vi "LoopselFF_1_or_2cam_eventdriven.VI"() -> ()   [LabVIEW 2015]
uses:
  board.vis/Globals.vi
  <vilib>/Analysis/NI_AALBase.lvlib
panel:
  out "tRMS":dbl=8.272957184592048 format="%0#.1f"
  out "mean":dbl=3064.5285285285286 format="%#_4f"
  in  "Pixel":u16=100
  in  "continuous":bool=TRUE
  out "curr.block":dbl=1.0
  out "Measure ON":bool
  in  "cam select\n1: cam 1\n2: cam 2\n3: both cams":u8=3
  in  "no.of blocks (nob)\npress enter":u32=1
  in  "NOB":u32(slide)=1 max=10 scale=0.9..1.0
  out "Signalverlaufgraph 2":u16[](graph)=[0, 0, 543, 543, 0, 1, 0, 0, 2, 2, 3, 3, 4, 4, 5, 5, 6, 6, 7, 7, 8, 8, 9, 9, 10, 10, 11, 11, 12, 12, 13, 13, 14, 14, 15, 15, 16, 16, 17, 17, 18, 18, 19, 19, 20, 20, 21, 21, 22, 22, 23, 23, 24, 24, 25, 25, 26, 26, 27, 27, 28, 28, 29, 29, 30, 30, 31, 31, 32, 32, 33, 33, 34, 34, 35, 35, 36, 36, 37, 37, 38, 38, 39, 39, 40, 40, 41, 41, 42, 42, 43, 43, 44, 44, 45, 45, 46, 46, 47, 47, 48, 48, 49, 49, 50, 50, 51, 51, 52, 52, 53, 53, 54, 54, 55, 55, 56, 56, 57, 57, 58, 58, 59, 59, 60, 60, 61, 61, 62, 62, 63, 63, 64, 64, 65, 65, 66, 66, 67, 67, 68, 68, 69, 69, 70, 70, 71, 71, 72, 72, 73, 73, 74, 74, 75, 75, 76, 76, 77, 77, 78, 78, 79, 79, 80, 80, 81, 81, 82, 82, 83, 83, 84, 84, 85, 85, 86, 86, 87, 87, 88, 88, 89, 89, 90, 90, 91, 91, 92, 92, 93, 93, 94, 94, 95, 95, 96, 96, 97, 97, 98, 98, 99, 99, 100, 100, 101, 101, 102, 102, 103, 103, 104, 104, 105, 105, 106, 106, 107, 107, 108, 108, 109, 109, 110, 110, 111, 111, 112, 112, 113, 113, 114, 114, 115, 115, 116, 116, 117, 117, 118, 118, 119, 119, 120, 120, 121, 121, 122, 122, 123, 123, 124, 124, 125, 125, 126, 126, 127, 127, 128, 128, 129, 129, 130, 130, 131, 131, 132, 132, 133, 133, 134, 134, 135, 135, 136, 136, 137, 137, 138, 138, 139, 139, 140, 140, 141, 141, 142, 142, 143, 143, 144, 144, 145, 145, 146, 146, 147, 147, 148, 148, 149, 149, 150, 150, 151, 151, 152, 152, 153, 153, 154, 154, 155, 155, 156, 156, 157, 157, 158, 158, 159, 159, 160, 160, 161, 161, 162, 162, 163, 163, 164, 164, 165, 165, 166, 166, 167, 167, 168, 168, 169, 169, 170, 170, 171, 171, 172, 172, 173, 173, 174, 174, 175, 175, 176, 176, 177, 177, 178, 178, 179, 179, 180, 180, 181, 181, 182, 182, 183, 183, 184, 184, 185, 185, 186, 186, 187, 187, 188, 188, 189, 189, 190, 190, 191, 191, 192, 192, 193, 193, 194, 194, 195, 195, 196, 196, 197, 197, 198, 198, 199, 199, 200, 200, 201, 201, 202, 202, 203, 203, 204, 204, 205, 205, 206, 206, 207, 207, 208, 208, 209, 209, 210, 210, 211, 211, 212, 212, 213, 213, 214, 214, 215, 215, 216, 216, 217, 217, 218, 218, 219, 219, 220, 220, 221, 221, 222, 222, 223, 223, 224, 224, 225, 225, 226, 226, 227, 227, 228, 228, 229, 229, 230, 230, 231, 231, 232, 232, 233, 233, 234, 234, 235, 235, 236, 236, 237, 237, 238, 238, 239, 239, 240, 240, 241, 241, 242, 242, 243, 243, 244, 244, 245, 245, 246, 246, 247, 247, 248, 248, 249, 249, 250, 250, 251, 251, 252, 252, 253, 253, 254, 254, 255, 255, 256, 256, 257, 257, 258, 258, 259, 259, 260, 260, 261, 261, 262, 262, 263, 263, 264, 264, 265, 265, 266, 266, 267, 267, 268, 268, 269, 269, 270, 270, 271, 271, 272, 272, 273, 273, 274, 274, 275, 275, 276, 276, 277, 277, 278, 278, 279, 279, 280, 280, 281, 281, 282, 282, 283, 283, 284, 284, 285, 285, 286, 286, 287, 287, 288, 288, 289, 289, 290, 290, 291, 291, 292, 292, 293, 293, 294, 294, 295, 295, 296, 296, 297, 297, 298, 298, 299, 299, 300, 300, 301, 301, 302, 302, 303, 303, 304, 304, 305, 305, 306, 306, 307, 307, 308, 308, 309, 309, 310, 310, 311, 311, 312, 312, 313, 313, 314, 314, 315, 315, 316, 316, 317, 317, 318, 318, 319, 319, 320, 320, 321, 321, 322, 322, 323, 323, 324, 324, 325, 325, 326, 326, 327, 327, 328, 328, 329, 329, 330, 330, 331, 331, 332, 332, 333, 333, 334, 334, 335, 335, 336, 336, 337, 337, 338, 338, 339, 339, 340, 340, 341, 341, 342, 342, 343, 343, 344, 344, 345, 345, 346, 346, 347, 347, 348, 348, 349, 349, 350, 350, 351, 351, 352, 352, 353, 353, 354, 354, 355, 355, 356, 356, 357, 357, 358, 358, 359, 359, 360, 360, 361, 361, 362, 362, 363, 363, 364, 364, 365, 365, 366, 366, 367, 367, 368, 368, 369, 369, 370, 370, 371, 371, 372, 372, 373, 373, 374, 374, 375, 375, 376, 376, 377, 377, 378, 378, 379, 379, 380, 380, 381, 381, 382, 382, 383, 383, 384, 384, 385, 385, 386, 386, 387, 387, 388, 388, 389, 389, 390, 390, 391, 391, 392, 392, 393, 393, 394, 394, 395, 395, 396, 396, 397, 397, 398, 398, 399, 399, 400, 400, 401, 401, 402, 402, 403, 403, 404, 404, 405, 405, 406, 406, 407, 407, 408, 408, 409, 409, 410, 410, 411, 411, 412, 412, 413, 413, 414, 414, 415, 415, 416, 416, 417, 417, 418, 418, 419, 419, 420, 420, 421, 421, 422, 422, 423, 423, 424, 424, 425, 425, 426, 426, 427, 427, 428, 428, 429, 429, 430, 430, 431, 431, 432, 432, 433, 433, 434, 434, 435, 435, 436, 436, 437, 437, 438, 438, 439, 439, 440, 440, 441, 441, 442, 442, 443, 443, 444, 444, 445, 445, 446, 446, 447, 447, 448, 448, 449, 449, 450, 450, 451, 451, 452, 452, 453, 453, 454, 454, 455, 455, 456, 456, 457, 457, 458, 458, 459, 459, 460, 460, 461, 461, 462, 462, 463, 463, 464, 464, 465, 465, 466, 466, 467, 467, 468, 468, 469, 469, 470, 470, 471, 471, 472, 472, 473, 473, 474, 474, 475, 475, 476, 476, 477, 477, 478, 478, 479, 479, 480, 480, 481, 481, 482, 482, 483, 483, 484, 484, 485, 485, 486, 486, 487, 487, 488, 488, 489, 489, 490, 490, 491, 491, 492, 492, 493, 493, 494, 494, 495, 495, 496, 496, 497, 497, 498, 498, 499, 499, 500, 500, 501, 501, 502, 502, 503, 503, 504, 504, 505, 505, 506, 506, 507, 507, 508, 508, 509, 509, 510, 510, 511, 511, 512, 512, 513, 513, 514, 514, 515, 515, 516, 516, 517, 517, 518, 518, 519, 519, 520, 520, 521, 521, 522, 522, 523, 523, 524, 524, 525, 525, 526, 526, 527, 527, 528, 528, 529, 529, 530, 530, 531, 531, 532, 532, 533, 533, 534, 534, 535, 535, 536, 536, 537, 537, 538, 538, 539, 539, 540, 540, 541, 541]
  out "Signalverlaufgraph":u16[](graph)=[2357, 2347, 2353, 2358, 0, 1, 0, 1, 2411, 2350, 2363, 2362, 2360, 34762, 35034, 35066, 35068, 35077, 35067, 35071, 35078, 35087, 35089, 35073, 35080, 35063, 35067, 35068, 35056, 35053, 35026, 35070, 35060, 35052, 35055, 35054, 35023, 35040, 35048, 35039, 35058, 35037, 35044, 35031, 35053, 35025, 35066, 35061, 35050, 35073, 35076, 35083, 35075, 35070, 35075, 35085, 35086, 35080, 35089, 35095, 35070, 35081, 35104, 35104, 35105, 35092, 35088, 35095, 35088, 35081, 35081, 35088, 35080, 35084, 35070, 35082, 35073, 35056, 35058, 35059, 35053, 35054, 35077, 35067, 35059, 35054, 35062, 35059, 35059, 35062, 35066, 35064, 35074, 35065, 35068, 35067, 35064, 35069, 35062, 35075, 35092, 35065, 35066, 35083, 35080, 35080, 35081, 35105, 35099, 35081, 35093, 35095, 35085, 35101, 35101, 35088, 35100, 35088, 35099, 35088, 35085, 35101, 35074, 35079, 35081, 35069, 35058, 35069, 35068, 35075, 35079, 35072, 35080, 35080, 35067, 35078, 35064, 35073, 35063, 35054, 35076, 35075, 35084, 35082, 35085, 35067, 35059, 35082, 35080, 35097, 35083, 35088, 35093, 35097, 35078, 35088, 35097, 35091, 35100, 35088, 35091, 35092, 35100, 35086, 35085, 35097, 35088, 35086, 35079, 35077, 35080, 35089, 35073, 35075, 35083, 35074, 35085, 35070, 35078, 35081, 35070, 35060, 35084, 35077, 35080, 35075, 35069, 35069, 35061, 35065, 35065, 35085, 35071, 35088, 35086, 35088, 35089, 35090, 35091, 35088, 35079, 35100, 35098, 35102, 35082, 35075, 35088, 35079, 35086, 35082, 35098, 35088, 35092, 35085, 35085, 35084, 35097, 35085, 35074, 35072, 35085, 35088, 35079, 35079, 35080, 35085, 35094, 35077, 35090, 35081, 35083, 35089, 35090, 35083, 35083, 35086, 35087, 35083, 35094, 35098, 35093, 35103, 35102, 35089, 35096, 35096, 35078, 35075, 35103, 35084, 35089, 35095, 35093, 35085, 35094, 35090, 35100, 35080, 35099, 35081, 35086, 35095, 35101, 35083, 35090, 35087, 35078, 35096, 35077, 35091, 35102, 35089, 35093, 35100, 35081, 35086, 35088, 35093, 35079, 35088, 35083, 35083, 35100, 35107, 35081, 35096, 35098, 35091, 35098, 35106, 35087, 35107, 35094, 35101, 35099, 35085, 35088, 35093, 35084, 35089, 35100, 35096, 35094, 35099, 35085, 35094, 35089, 35104, 35088, 35103, 35099, 35088, 35088, 35083, 35092, 35097, 35096, 35095, 35098, 35076, 35100, 35091, 35084, 35090, 35100, 35110, 35101, 35071, 35094, 35088, 35097, 35076, 35103, 35100, 35102, 35101, 35094, 35096, 35103, 35088, 35093, 35099, 35099, 35102, 35099, 35104, 35089, 35085, 35094, 35110, 35093, 35109, 35094, 35101, 35088, 35100, 35090, 35088, 35090, 35086, 35093, 35107, 35091, 35099, 35104, 35088, 35093, 35093, 35098, 35097, 35108, 35087, 35107, 35092, 35094, 35098, 35097, 35092, 35093, 35085, 35095, 35102, 35094, 35093, 35115, 35088, 35106, 35079, 35105, 35099, 35091, 35128, 35094, 35089, 35088, 35109, 35110, 35087, 35110, 35096, 35095, 35097, 35091, 35099, 35085, 35087, 35112, 35089, 35102, 35085, 35089, 35106, 35094, 35097, 35113, 35110, 35087, 35105, 35097, 35094, 35097, 35097, 35098, 35112, 35092, 35101, 35106, 35092, 35094, 35085, 35107, 35088, 35089, 35094, 35081, 35094, 35103, 35107, 35097, 35101, 35086, 35094, 35108, 35086, 35098, 35102, 35102, 35096, 35080, 35085, 35100, 35089, 35088, 35104, 35112, 35100, 35102, 35102, 35097, 35106, 35099, 35081, 35097, 35101, 35109, 35100, 35114, 35098, 35092, 32940, 29697, 29585, 29528, 29434, 29346, 29303, 29248, 29143, 29102, 29112, 29035, 28966, 28956, 28848, 28789, 28725, 28651, 28612, 28562, 28516, 28427, 28371, 28320, 28264, 28200, 28178, 28101, 28056, 27957, 27925, 27901, 27776, 27758, 27701, 27631, 27579, 27545, 27475, 27425, 27382, 27318, 27302, 27222, 27176, 27114, 27069, 27020, 26974, 26944, 26887, 26793, 26807, 26744, 26714, 26624, 26586, 26540, 26466, 26393, 26379, 26282, 26220, 26157, 26029, 25929, 25768, 25543, 2252, 2400, 2386, 2390, 2368, 2373, 2377, 2379, 2379, 2378, 2377, 2380, 2373, 2379, 2386, 2383, 2376, 2381, 2378, 2377, 2376, 2373, 2385, 2377, 2381, 2376, 2379, 2379, 2376, 2376, 2376, 2379, 2384, 2378, 2374, 2380, 2377, 2381, 2380, 2371, 2379, 2376, 2379, 2384, 2380, 2380, 2377, 2368, 2376, 2375, 2378, 2370, 2374, 2375, 2383, 2372, 2379, 2374, 2381, 2369, 2375, 2368, 2373, 2368, 2368, 2372, 2374, 2371, 2368, 2373, 2372, 2370, 2372, 2374, 2375, 2367, 2367, 2370, 2369, 2375, 2372, 2373, 2378, 2372, 2366, 2372, 2370, 2374, 2365, 2373, 2375, 2374, 2370, 2370, 2369, 2369, 2374, 2371, 2373, 2371, 2372, 2371, 2366, 2368, 2370, 2362, 2370, 2372, 2366, 2374, 2369, 2368, 2371, 2368, 2365, 2362, 2375, 2373, 2369, 2366, 2367, 2371, 2362, 2377, 2371, 2367, 2369, 2366, 2371, 2366, 2364, 2366, 2360, 2365, 2374, 2362, 2371, 2373, 2366, 2364, 2367, 2364, 2368, 2360, 2360, 2363, 2367, 2368, 2367, 2371, 2364, 2368, 2366, 2359, 2363, 2365, 2368, 2368, 2358, 2357, 2365, 2364, 2369, 2362, 2364, 2364, 2363, 2358, 2363, 2364, 2359, 2360, 2358, 2370, 2358, 2361, 2363, 2355, 2361, 2369, 2363, 2366, 2365, 2368, 2363, 2360, 2359, 2361, 2359, 2363, 2356, 2365, 2362, 2360, 2368, 2362, 2366, 2370, 2358, 2366, 2364, 2366, 2362, 2363, 2356, 2365, 2363, 2361, 2363, 2367, 2366, 2365, 2357, 2366, 2359, 2361, 2360, 2360, 2363, 2365, 2364, 2360, 2360, 2357, 2355, 2362, 2361, 2361, 2364, 2364, 2361, 2364, 2361, 2363, 2358, 2363, 2357, 2355, 2357, 2365, 2357, 2367, 2365, 2363, 2354, 2360, 2356, 2358, 2362, 2359, 2360, 2362, 2362, 2355, 2360, 2360, 2360, 2361, 2360, 2359, 2357, 2364, 2359, 2361, 2362, 2360, 2359, 2360, 2355, 2355, 2362, 2358, 2358, 2357, 2357, 2360, 2360, 2363, 2353, 2353, 2358, 2358, 2358, 2362, 2360, 2362, 2359, 2356, 2357, 2360, 2355, 2353, 2360, 2362, 2358, 2358, 2350, 2357, 2362, 2354, 2354, 2356, 2360, 2360, 2355, 2361, 2354, 2360, 2356, 2355, 2355, 2362, 2359, 2362, 2363, 2359, 2361, 2358, 2355, 2356, 2354, 2358, 2364, 2356, 2362, 2358, 2354, 2360, 2362, 2361, 2358, 2361, 2362, 2358, 2363, 2359, 2363, 2364, 2356, 2357, 2356, 2354, 2360, 2357, 2355, 2359, 2358, 2356, 2362, 2360, 2357, 2359, 2357, 2357, 2355, 2357, 2357, 2357, 2364, 2360, 2355, 2358, 2355, 2357, 2360, 2353, 2355, 2352, 2362, 2354, 2355, 2360, 2357, 2352, 2359, 2356, 2356, 2358, 2353, 2357, 2356, 2355, 2349, 2361, 2358, 2354, 2358, 2359, 2355, 2360, 2354, 2357, 2357, 2353, 2354, 2359, 2359, 2355, 2349, 2358, 2358, 2355, 2353, 2353, 2357, 2357, 2357, 2354, 2358, 2359, 2354, 2353, 2352, 2358, 2361, 2357, 2350, 2350, 2352, 2360, 2351, 2355, 2354, 2360, 2357, 2355, 2355, 2355, 2350, 2357, 2357, 2358, 2358, 2356, 2353, 2352, 2354, 2353, 2357, 2357, 2353, 2358, 2360, 2361, 2355, 2357, 2361, 2357, 2358, 2356, 2355, 2358, 2354, 2351, 2355, 2352, 2354, 2352, 2354, 2363, 2359, 2358, 2357, 2349, 2358, 2352, 2356, 2355, 2359, 2353, 2353, 2361, 2359, 2359, 2357, 2357, 2349, 2353, 2353, 2350, 2358, 2357, 2356, 2358, 2356, 2356, 2355, 2355, 2355, 2351, 2355, 2357, 2352, 2354, 2348, 2354, 2348, 2354, 2350, 2352, 2353, 2359, 2356, 2351, 2356, 2357, 2352, 2354, 2355, 2359, 2353, 2354, 2352, 2349, 2362, 2353, 2360, 2349, 2357, 2352, 2359, 2348, 2359, 2349, 2358, 2348, 2349, 2351, 2356, 2353, 2358, 2353, 2354, 2360, 2355, 2356, 2358, 2348, 2351, 2354, 2358, 2360, 2360, 2359, 2356, 2356, 2354, 2357, 2350, 2351, 2351]
  out "cams recognised":u8=1
  in  "alloc mem":bool
  out "FREE \nRAM MB":u64=14941
  out "BUILT-IN\nRAM MB":u64=18096
  out "SEC":dbl=5.9999999999999995e-05
  out "MB RAM":u64
  in  "pos slope":u8=1
  in  "both slopes":u8
  in  "DAT in 10ns":u32
  in  "extTrig  0/1\n0 : internal\n1:  \"I\" input (laser)":u8
  in  "stop all":bool
  in  "start":bool
  in  "NOS":u32(slide)=2 max=3000 scale=0.9..1000.0
  in  "no.of samples (nos)":u32=3
  in  "exposuretime[ms]":dbl=1.0 format="%.3f"
  # "Start with run"
  # "Abort with ESC"
  # "press Esc to stop measurement"
  # "exit here"
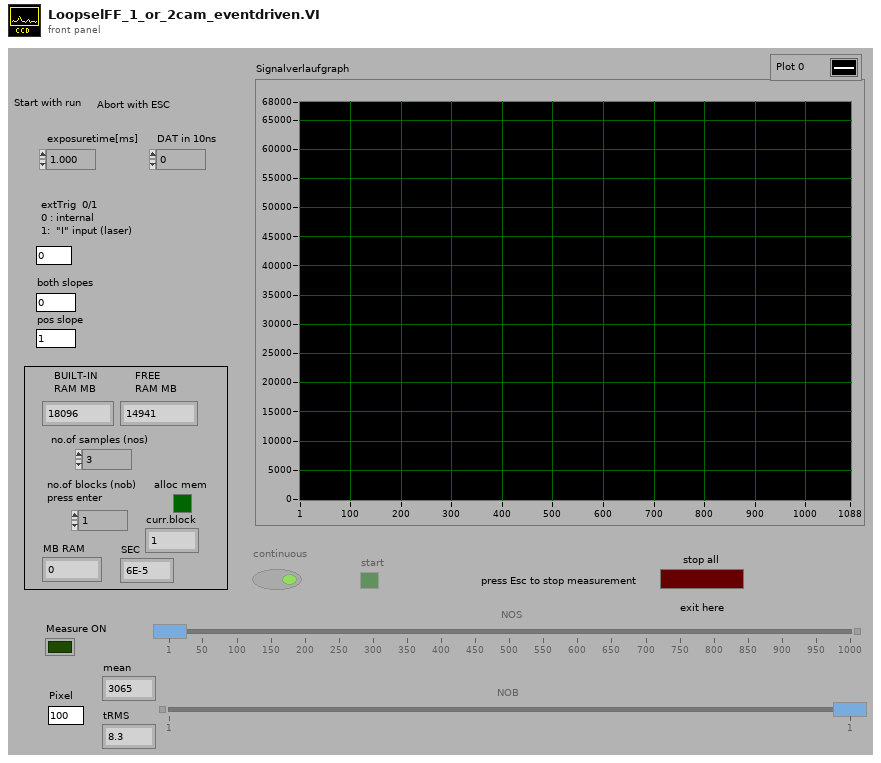
[diagram p1: front panel]
types:
  T1 = enum8{"Enabled", "Disabled", "Disabled and Grayed Out"}
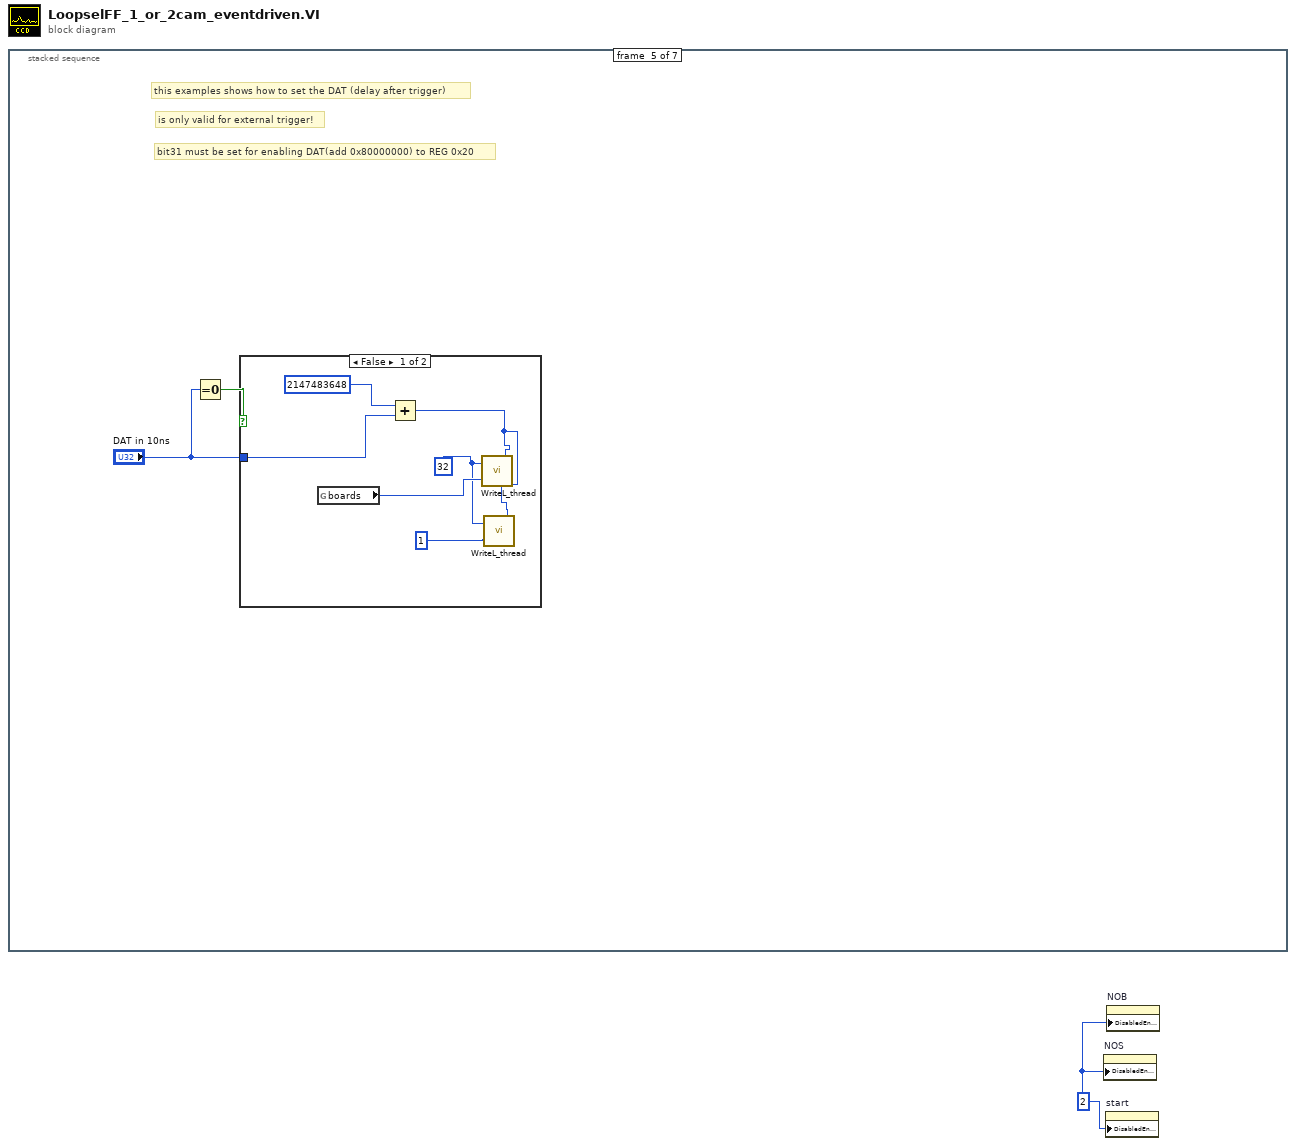
[diagram p0: block diagram]
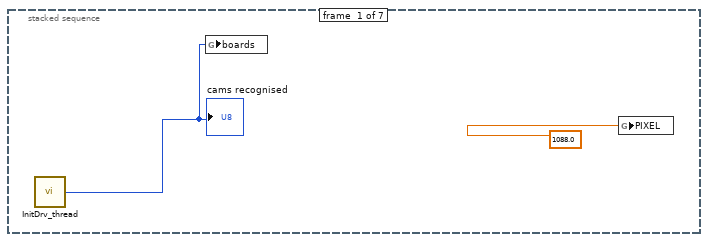
[diagram p2: hidden frame]
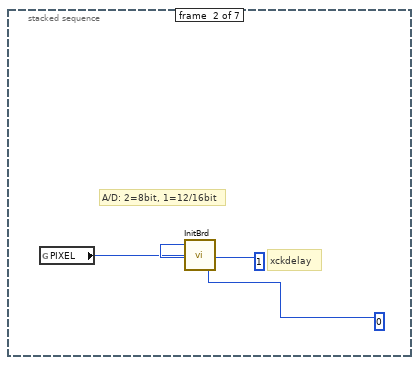
[diagram p3: hidden frame]
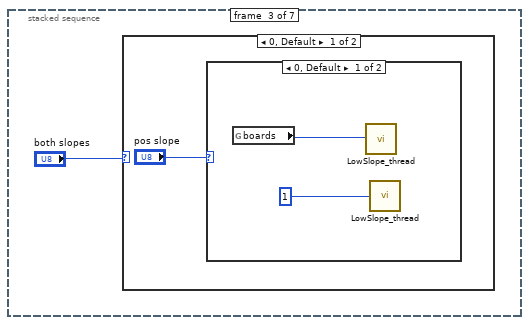
[diagram p4: hidden frame]
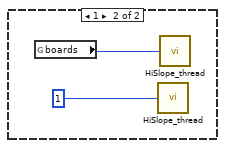
[diagram p5: hidden frame]
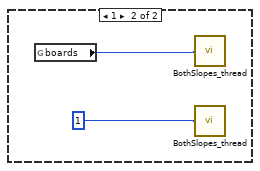
[diagram p6: hidden frame]
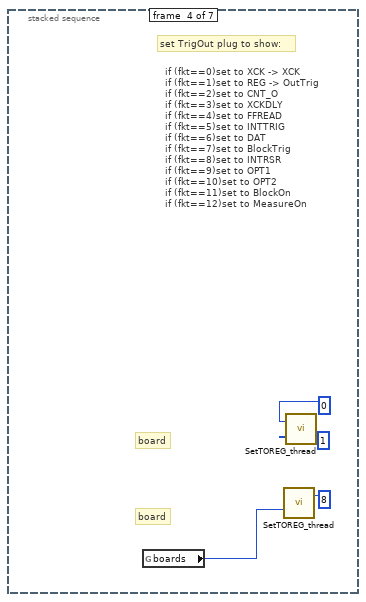
[diagram p7: hidden frame]
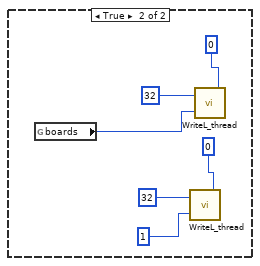
[diagram p8: hidden frame]
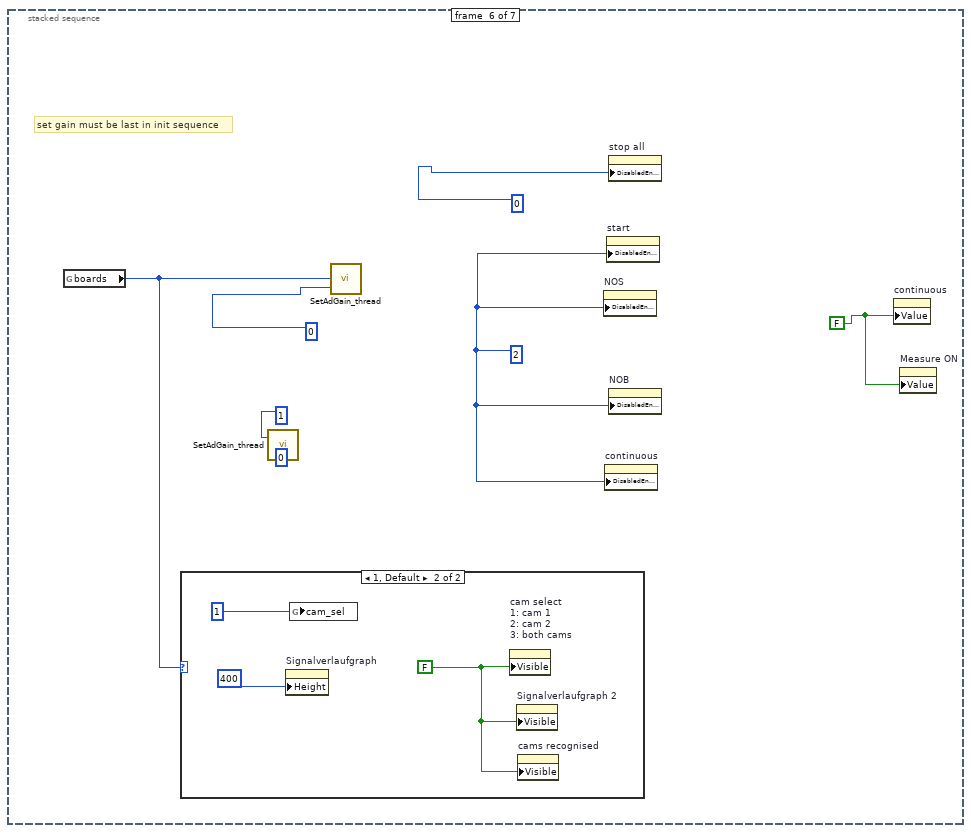
[diagram p9: hidden frame]
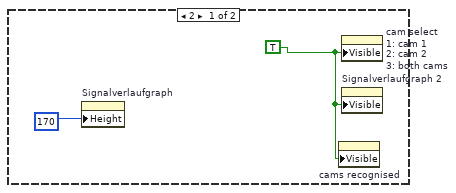
[diagram p10: hidden frame]
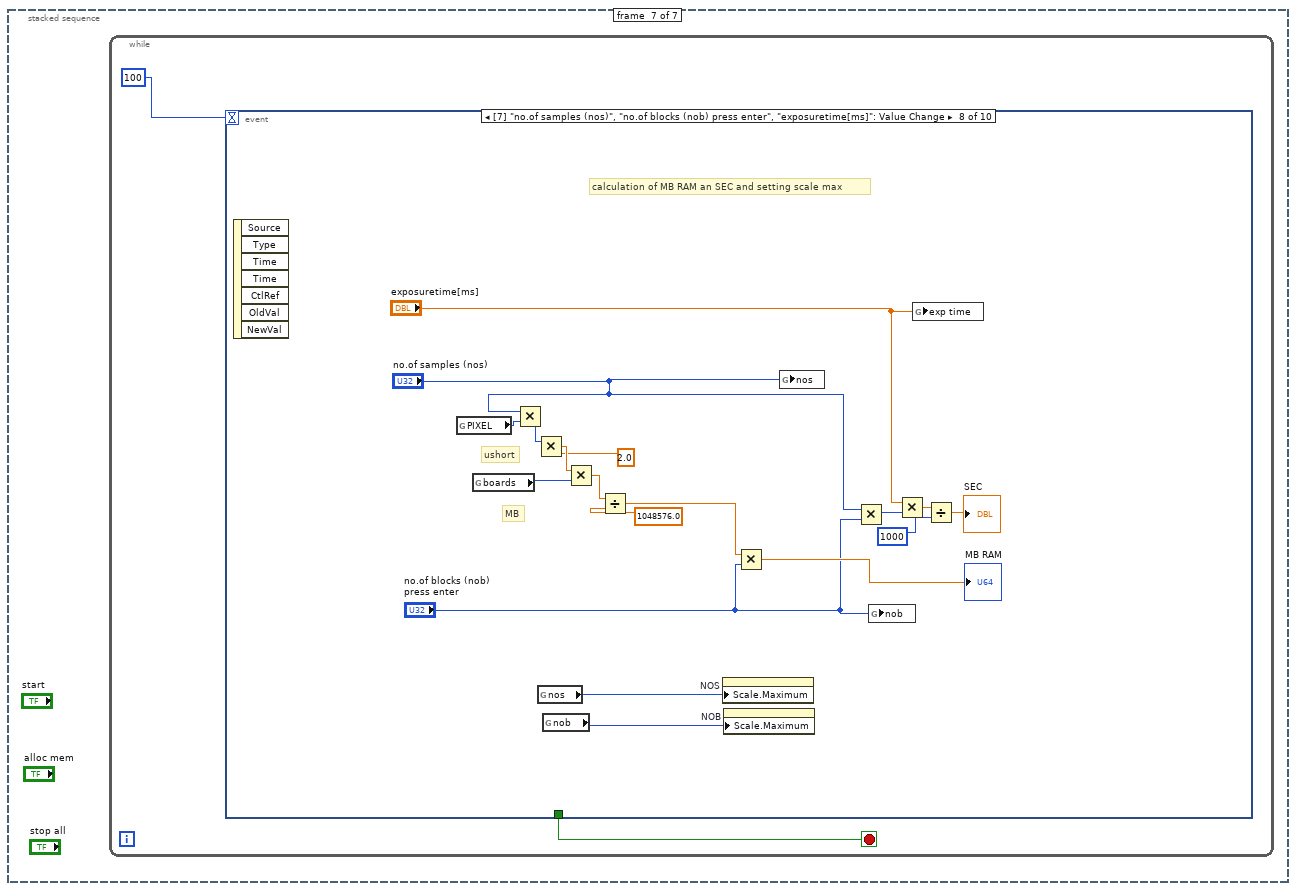
[diagram p11: hidden frame]
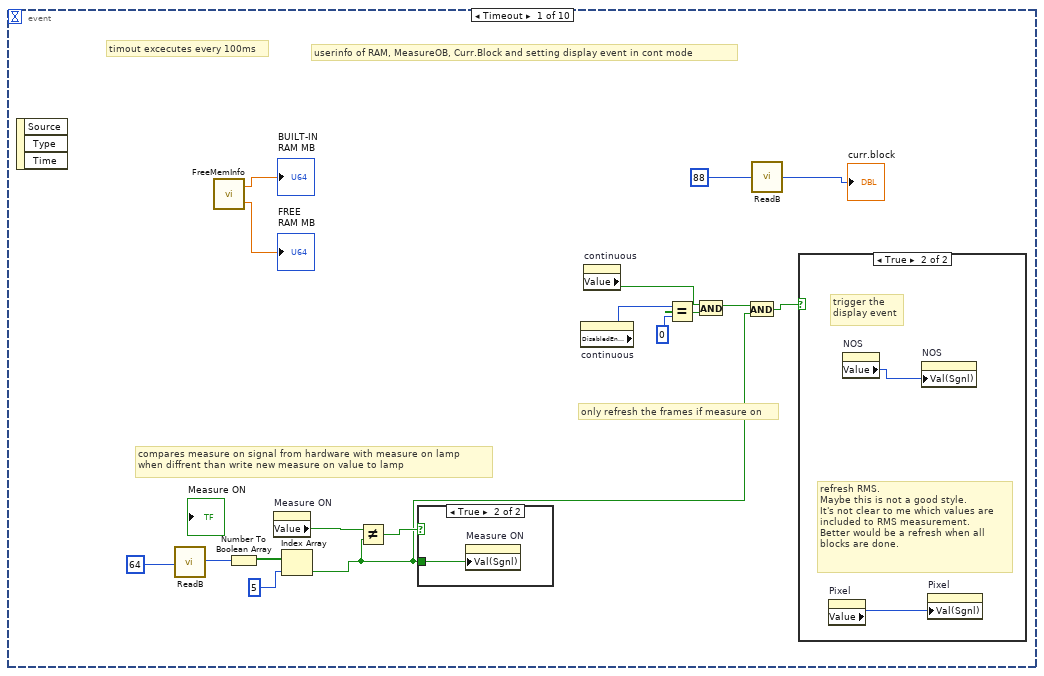
[diagram p12: hidden frame]
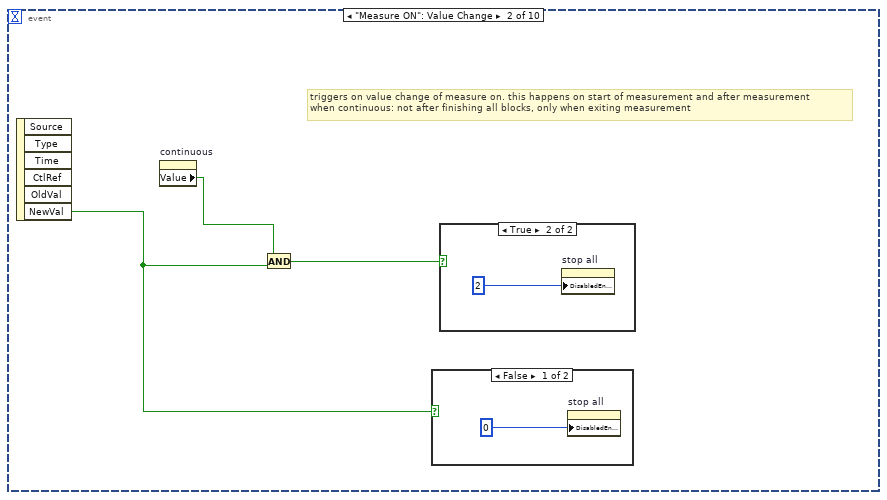
[diagram p15: hidden frame]
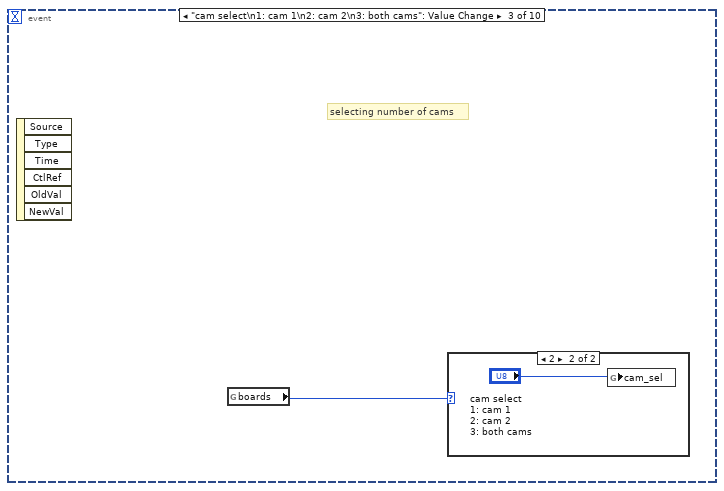
[diagram p18: hidden frame]
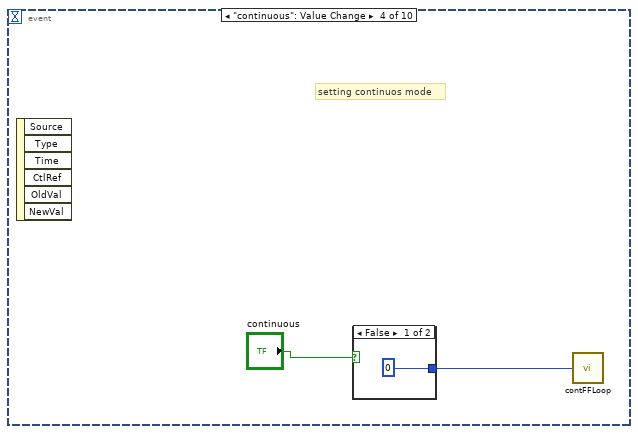
[diagram p20: hidden frame]
diagram:
  w1 = 2
  n1 = stacked-sequence {
    frame #0 {
      n2 = call "InitDrv_thread.vi"() -> ("Boards"=w2:u8)  [unwired: 1 in]
      "cams recognised" <- w2
      n3 = global write "Globals.vi" "boards"(w2) -> ()
      n4 = global write "Globals.vi" "PIXEL"(1088.0) -> ()
    }
    frame #1 {
      # "xckdelay"
      # "A/D: 2=8bit, 1=12/16bit"
      n5 = global read "Globals.vi" "PIXEL"() -> (w4:u32)
      n6 = call "InitBrd.vi"("xckdly"=u32 0, "pixel"=w4, "flag816"=u32 1) -> ()  [unwired: 3 in]
    }
    frame #2 {
      n7 = case shown="0, Default" "both slopes" {
        frame 0, Default {
          n8 = case shown="0, Default" "pos slope" {
            frame 0, Default {
              n9 = global read "Globals.vi" "boards"() -> (w9:u32)
              n10 = call "LowSlope_thread.vi"("board"=w9) -> ()  [unwired: 1 in]
              n11 = call "LowSlope_thread.vi"("board"=1) -> ()  [unwired: 1 in]
            }
            frame 1 {
              n12 = global read "Globals.vi" "boards"() -> (w12:u32)
              n13 = call "HiSlope_thread.vi"("board"=1) -> ()  [unwired: 1 in]
              n14 = call "HiSlope_thread.vi"("board"=w12) -> ()  [unwired: 1 in]
            }
          }
        }
        frame 1 {
          n15 = global read "Globals.vi" "boards"() -> (w14:u32)
          n16 = call "BothSlopes_thread.vi"("board"=w14) -> ()  [unwired: 1 in]
          n17 = call "BothSlopes_thread.vi"("board"=1) -> ()  [unwired: 1 in]
        }
      }
    }
    frame #3 {
      # "board"
      # "board"
      # "set TrigOut plug to show:"
      # "if (fkt==0)set to XCK -> XCK\nif (fkt==1)set to REG -> OutTrig\nif (fkt==2)set to CNT_O\nif (fkt==3)set to XCKDLY\nif (fkt==4)set to FFREAD\nif (fkt==5)set to INTTRIG\nif (fkt==6)set to DAT\nif (fkt==7)set to BlockTrig\nif (fkt==8)set to INTRSR\nif (fkt==9)set to OPT1\nif (fkt==10)set to OPT2\nif (fkt==11)set to BlockOn\nif (fkt==12)set to MeasureOn"
      n18 = global read "Globals.vi" "boards"() -> (w18:u32)
      n19 = call "SetTOREG_thread.vi"("board"=w18, "fkt"=u8 8) -> ()  [unwired: 1 in]
      n20 = call "SetTOREG_thread.vi"("board"=u8 1, "fkt"=u8 0) -> ()  [unwired: 1 in]
    }
    frame #4 {
      # "bit31 must be set for enabling DAT(add 0x80000000) to REG 0x20"
      # "is only valid for external trigger!"
      # "this examples shows how to set the DAT (delay after trigger)"
      n21 = Equal To 0?(x="DAT in 10ns") -> (x = 0?=w20:bool)
      n22 = case shown="False" w20 {
        tunnel: "DAT in 10ns" -> [w25 _]
        frame False {
          w22 = u32 32
          n23 = global read "Globals.vi" "boards"() -> (w24:u32)
          n24 = Add(x=u32 2147483648, y=w25) -> (x+y=w23:u32)
          n25 = call "WriteL_thread.vi"("val"=w23, "board"=w24, "offset"=w22) -> ()
          n26 = call "WriteL_thread.vi"("val"=w23, "board"=1, "offset"=w22) -> ()
        }
        frame True {
          n27 = global read "Globals.vi" "boards"() -> (w31:u32)
          n28 = call "WriteL_thread.vi"("val"=0, "board"=1, "offset"=u32 32) -> ()
          n29 = call "WriteL_thread.vi"("val"=0, "board"=w31, "offset"=u32 32) -> ()
        }
      }
    }
    frame #5 {
      w33 = FALSE
      w39 = 2
      # "set gain must be last in init sequence"
      n30 = global read "Globals.vi" "boards"() -> (w37:u32)
      n31 = case shown="1, Default" w37 {
        frame 2 {
          w41 = TRUE
          n32 = property on="Signalverlaufgraph" class="WFGraph (strict)"("Height"=u8 170) -> ()  [unwired: 2 in, 2 out]
          n33 = property on="cams recognised" class="DigNum (strict)"("Visible"=w41) -> ()  [unwired: 2 in, 2 out]
          n34 = property on="cam select\n1: cam 1\n2: cam 2\n3: both cams" class="DigNum (strict)"("Visible"=w41) -> ()  [unwired: 2 in, 2 out]
          n35 = property on="Signalverlaufgraph 2" class="WFGraph (strict)"("Visible"=w41) -> ()  [unwired: 2 in, 2 out]
        }
        frame 1, Default {
          w42 = FALSE
          n36 = property on="Signalverlaufgraph" class="WFGraph (strict)"("Height"=400) -> ()  [unwired: 2 in, 2 out]
          n37 = global write "Globals.vi" "cam_sel"(u8 1) -> ()
          n38 = property on="cam select\n1: cam 1\n2: cam 2\n3: both cams" class="DigNum (strict)"("Visible"=w42) -> ()  [unwired: 2 in, 2 out]
          n39 = property on="Signalverlaufgraph 2" class="WFGraph (strict)"("Visible"=w42) -> ()  [unwired: 2 in, 2 out]
          n40 = property on="cams recognised" class="DigNum (strict)"("Visible"=w42) -> ()  [unwired: 2 in, 2 out]
        }
      }
      n41 = call "SetAdGain_thread.vi"("gain"=u8 0, "board"=u32 1) -> ()  [unwired: 1 in]
      n42 = call "SetAdGain_thread.vi"("gain"=u8 0, "board"=w37) -> ()  [unwired: 1 in]
      n43 = property on="NOS" class="Slide (strict)"("DisabledEnum"=w39) -> ()  [unwired: 2 in, 2 out]
      n44 = property on="continuous" class="Bool (strict)"("DisabledEnum"=w39) -> ()  [unwired: 2 in, 2 out]
      n45 = property on="start" class="Bool (strict)"("DisabledEnum"=w39) -> ()  [unwired: 2 in, 2 out]
      n46 = property on="stop all" class="Bool (strict)"("DisabledEnum"=0) -> ()  [unwired: 2 in, 2 out]
      n47 = property on="NOB" class="Slide (strict)"("DisabledEnum"=w39) -> ()  [unwired: 2 in, 2 out]
      n48 = property on="continuous" class="Bool (strict)"("Value"=w33) -> ()  [unwired: 2 in, 2 out]
      n49 = property on="Measure ON" class="Bool (strict)"("Value"=w33) -> ()  [unwired: 2 in, 2 out]
    }
    frame #6 {
      n50 = while {
        stop <- w46 stop-if-true
        n51 = event shown="[7] \"no.of samples (nos)\", \"no.of blocks (nob) press enter\", \"exposuretime[ms]\": Value Change" {
          selector: _ -> [_ _ _ _ _ _ _ _ _ _]
          dyn-events: _ -> [_ _ _ _ _ _ _ _ _ _]
          timeout: 100 -> [_ _ _ _ _ _ _ _ _ _]
          tunnel: [_ _ _ _ _ _ _ _ w141 _] -> w46
          event Timeout {
            # "only refresh the frames if measure on"
            # "compares measure on signal from hardware with measure on lamp\nwhen diffrent than write new measure on value to lamp"
            # "timout excecutes every 100ms"
            # "userinfo of RAM, MeasureOB, Curr.Block and setting display event in cont mode"
            n52 = event-data() -> ()  [unwired: 1 in, 3 out]
            n53 = call "ReadB.vi"("Offset"=64) -> ("Data"=w60:u8)
            n54 = call "FreeMemInfo.vi"() -> ("PhysicalSpace"=→"BUILT-IN\nRAM MB":dbl, "PhysicalFreeSpace"=→"FREE \nRAM MB":dbl)  [unwired: 1 in]
            n55 = Number To Boolean Array(number=w60) -> (Boolean array=w59:bool[])
            n56 = property on="Measure ON" class="Bool (strict)"() -> ("Value"=w51:bool)  [unwired: 2 in, 2 out]
            n57 = Index Array(array=w59, index=5) -> (element=w47:bool)
            n58 = Not Equal?(x=w51, y=w47) -> (x != y?=w50:bool)
            n59 = case shown="True" w50 {
              tunnel: w47 -> [_ w64]
              frame False {
              }
              frame True {
                n60 = property on="Measure ON" class="Bool (strict)"("Val(Sgnl)"=w64) -> ()  [unwired: 2 in, 2 out]
              }
            }
            n61 = property on="continuous" class="Bool (strict)"() -> ("DisabledEnum"=w53:T1)  [unwired: 2 in, 2 out]
            n62 = property on="continuous" class="Bool (strict)"() -> ("Value"=w55:bool)  [unwired: 2 in, 2 out]
            n63 = Equal?(x=w53, y=0) -> (x = y?=w54:bool)
            n64 = And(x=w55, y=w54) -> (x .and. y?=w49:bool)
            n65 = And(x=w49, y=w47) -> (x .and. y?=w48:bool)
            n66 = call "ReadB.vi"("Offset"=88) -> ("Data"=→"curr.block":u8)
            n67 = case shown="True" w48 {
              frame False {
              }
              frame True {
                # "refresh RMS.\nMaybe this is not a good style.\nIt's not clear to me which values are \nincluded to RMS measurement.\nBetter would be a refresh when all\nblocks are done."
                # "trigger the \ndisplay event"
                n68 = property on="Pixel" class="DigNum (strict)"() -> ("Value"=w65:u16)  [unwired: 2 in, 2 out]
                n69 = property on="NOS" class="Slide (strict)"() -> ("Value"=w66:u32)  [unwired: 2 in, 2 out]
                n70 = property on="NOS" class="Slide (strict)"("Val(Sgnl)"=w66) -> ()  [unwired: 2 in, 2 out]
                n71 = property on="Pixel" class="DigNum (strict)"("Val(Sgnl)"=w65) -> ()  [unwired: 2 in, 2 out]
              }
            }
          }
          event "Measure ON": Value Change {
            # "triggers on value change of measure on. this happens on start of measurement and after measurement\nwhen continuous: not after finishing all blocks, only when exiting measurement"
            n72 = event-data() -> ("NewVal"=w67:bool)  [unwired: 1 in, 5 out]
            n73 = property on="continuous" class="Bool (strict)"() -> ("Value"=w68:bool)  [unwired: 2 in, 2 out]
            n74 = And(x=w68, y=w67) -> (x .and. y?=w69:bool)
            n75 = case shown="False" w67 {
              frame False {
                n76 = property on="stop all" class="Bool (strict)"("DisabledEnum"=0) -> ()  [unwired: 2 in, 2 out]
              }
              frame True {
              }
            }
            n77 = case shown="True" w69 {
              frame False {
              }
              frame True {
                n78 = property on="stop all" class="Bool (strict)"("DisabledEnum"=2) -> ()  [unwired: 2 in, 2 out]
              }
            }
          }
          event "cam select\n1: cam 1\n2: cam 2\n3: both cams": Value Change {
            # "selecting number of cams"
            n79 = event-data() -> ()  [unwired: 1 in, 6 out]
            n80 = global read "Globals.vi" "boards"() -> (w72:u32)
            n81 = case shown="2" w72 {
              frame 0, Default {
              }
              frame 2 {
                n82 = global write "Globals.vi" "cam_sel"("cam select\n1: cam 1\n2: cam 2\n3: both cams") -> ()
              }
            }
          }
          event "continuous": Value Change {
            # "setting continuos mode"
            n83 = event-data() -> ()  [unwired: 1 in, 6 out]
            n84 = case shown="False" "continuous" {
              tunnel: [0 1] -> w74
              frame False {
              }
              frame True {
              }
            }
            n85 = call "contFFLoop.vi"("Numeric"=w74) -> ()  [unwired: 1 in]
          }
          event "alloc mem": Value Change {
            w82 = 0
            # "update params"
            # "Setup DMA"
            n86 = event-data() -> ()  [unwired: 1 in, 6 out]
            n87 = global read "Globals.vi" "nob"() -> (w80:u32)
            n88 = global read "Globals.vi" "boards"() -> (w83:u32)
            n89 = global read "Globals.vi" "nos"() -> (w79:u32)
            n90 = case shown="2" w83 {
              selector: w83 -> [_ w84]
              tunnel: w79 -> [_ w85]
              tunnel: w80 -> [_ w86]
              frame 1, Default {
              }
              frame 2 {
                # "Setup DMA"
                n91 = call "SetupDMA_thread.vi"("blocks"=w86, "nos"=w85, "Drv"=w84) -> ()  [unwired: 2 in]
              }
            }
            n92 = call "SetupDMA_thread.vi"("blocks"=w80, "nos"=w79, "Drv"=u32 1) -> ()  [unwired: 2 in]
            n93 = property on="continuous" class="Bool (strict)"("DisabledEnum"=w82) -> ()  [unwired: 2 in, 2 out]
            n94 = property on="NOB" class="Slide (strict)"("DisabledEnum"=w82) -> ()  [unwired: 2 in, 2 out]
            n95 = property on="NOS" class="Slide (strict)"("DisabledEnum"=w82) -> ()  [unwired: 2 in, 2 out]
            n96 = property on="exposuretime[ms]" class="DigNum (strict)"() -> ("Value"=w81:dbl)  [unwired: 2 in, 2 out]
            n97 = property on="start" class="Bool (strict)"("DisabledEnum"=w82) -> ()  [unwired: 2 in, 2 out]
            n98 = property on="exposuretime[ms]" class="DigNum (strict)"("Val(Sgnl)"=w81) -> ()  [unwired: 2 in, 2 out]
          }
          event "start": Mouse Down {
            # "start measurement"
            # "only 1st PCI board is used for ext. trig."
            # "ext. block trig\n0: internal: Space\n1: PCI \"I\"\n2: S1\n3: S2"
            # "block trigger 0/1\n0: internal -> next block is started immediately \n1: external -> each block has an own trigger"
            n99 = event-data() -> ()  [unwired: 1 in, 8 out]
            n100 = global read "Globals.vi" "exp time"() -> (w92:dbl)
            n101 = Multiply(x=1000.0, y=w92) -> (x*y=w94:dbl)
            n102 = global read "Globals.vi" "cam_sel"() -> (w87:u8)
            n103 = To Unsigned Long Integer(number=w94) -> (unsigned 32bit integer=w89:u32)
            n104 = call "ReadFFLoop_thread.vi"("blocktrigger"=u8 0, "btrig_ch"=u8 0, "ExtTrig"="extTrig  0/1\n0 : internal\n1:  \"I\" input (laser)", "cam_sel"=w87, "exptus"=w89) -> ()  [unwired: 1 in]
          }
          event "NOS", "NOB": Value Change {
            w104 = 1
            # "when selecting a value\nbigger than possible\nnos or nob, a dummy \nvalue \"1\" is chosen\n\nTODO:\ninsert error handling\nwith lower values than 1"
            # "display"
            n105 = event-data() -> ()  [unwired: 1 in, 6 out]
            n106 = global read "Globals.vi" "boards"() -> (w107:u32)
            n107 = global read "Globals.vi" "nob"() -> (w96:u32)
            n108 = global read "Globals.vi" "nos"() -> (w103:u32)
            n109 = Greater?(x=w96, y="NOB") -> (0:w99:bool)
            n110 = Greater?(x=w103, y="NOS") -> (0:w102:bool)
            n111 = global read "Globals.vi" "PIXEL"() -> (w111:u32)
            n112 = case shown="True" w99 {
              tunnel: [1 w113] -> w98
              tunnel: "NOB" -> [_ w113]
              frame False {
              }
              frame True {
              }
            }
            n113 = case shown="False" w102 {
              tunnel: [1 w115] -> w101
              tunnel: "NOS" -> [_ w115]
              frame False {
              }
              frame True {
              }
            }
            n114 = Initialize Array(100, w111) -> (w110:i32[])
            n115 = Subtract(x=w101, y=w104) -> (x-y=w106:u32)
            n116 = Subtract(x=w98, y=w104) -> (x-y=w105:u32)
            n117 = case shown="2" w107 {
              selector: w107 -> [_ w118]
              tunnel: w106 -> [_ w119]
              tunnel: w105 -> [_ w116]
              frame 0, Default {
              }
              frame 2 {
                n118 = global read "Globals.vi" "PIXEL"() -> (w122:u32)
                n119 = Initialize Array(100, w122) -> (w121:i32[])
                n120 = call "ReturnFrame.vi"("Data Values In"=w121, "curr_nob"=w116, "curr_nos"=w119, "Drv"=w118) -> ("Data Values Out"=→"Signalverlaufgraph 2":u16[])  [unwired: 1 in]
              }
            }
            n121 = call "ReturnFrame.vi"("Data Values In"=w110, "curr_nob"=w105, "curr_nos"=w106, "Drv"=1) -> ("Data Values Out"=→"Signalverlaufgraph":u16[])  [unwired: 1 in]
          }
          event "no.of samples (nos)", "no.of blocks (nob)\npress enter", "exposuretime[ms]": Value Change {
            # "calculation of MB RAM an SEC and setting scale max"
            # "MB"
            # "ushort"
            n122 = event-data() -> ()  [unwired: 1 in, 7 out]
            n123 = global read "Globals.vi" "PIXEL"() -> (w140:u32)
            n124 = global read "Globals.vi" "boards"() -> (w139:u32)
            n125 = Multiply(x="no.of samples (nos)", y=w140) -> (x*y=w136:u32)
            n126 = Multiply(x=w136, y=2.0) -> (x*y=w137:dbl)
            n127 = global read "Globals.vi" "nos"() -> (w123:u32)
            n128 = global read "Globals.vi" "nob"() -> (w124:u32)
            n129 = Multiply(x=w137, y=w139) -> (x*y=w138:dbl)
            n130 = Divide(x=w138, y=1048576.0) -> (x/y=w128:dbl)
            n131 = property on="NOS" class="Slide (strict)"("Scale.Maximum"=w123) -> ()  [unwired: 2 in, 2 out]
            n132 = property on="NOB" class="Slide (strict)"("Scale.Maximum"=w124) -> ()  [unwired: 2 in, 2 out]
            n133 = Multiply(x=w128, y="no.of blocks (nob)\npress enter") -> (x*y=→"MB RAM":dbl)
            n134 = global write "Globals.vi" "nos"("no.of samples (nos)") -> ()
            n135 = Multiply(x="no.of samples (nos)", y="no.of blocks (nob)\npress enter") -> (x*y=w127:u32)
            n136 = global write "Globals.vi" "nob"("no.of blocks (nob)\npress enter") -> ()
            n137 = Multiply(x="exposuretime[ms]", y=w127) -> (x*y=w134:dbl)
            n138 = global write "Globals.vi" "exp time"("exposuretime[ms]") -> ()
            n139 = Divide(x=w134, y=1000) -> (x/y=→"SEC":dbl)
          }
          event "stop all": Value Change {
            # "exit"
            n140 = event-data() -> ()  [unwired: 1 in, 6 out]
            n141 = stacked-sequence {
              tunnel: [_ TRUE] -> w141
              frame #0 {
                n142 = call "FFStop.vi"() -> ()  [unwired: 1 in]
              }
              frame #1 {
                # "do not omit, or next call of driver will go wrong."
                n143 = call "Exit.vi"() -> ()  [unwired: 1 in]
              }
            }
          }
          event "Pixel": Value Change {
            # "one array with all values (except first 10)\nat index Pixel from all blocks"
            n144 = event-data() -> ()  [unwired: 1 in, 6 out]
            n145 = global read "Globals.vi" "nos"() -> (w146:u32)
            n146 = global read "Globals.vi" "nob"() -> (w147:u32)
            n147 = for {
              N: w147 -> [_]
              tunnel: w146 -> [w152]
              tunnel: [w148] -> w143 mode=concatenating
              i -> [w153]
              # "delete first 10 values"
              # "array of all values\nat index Pixel"
              n148 = for {
                N: w152 -> [_]
                tunnel: w153 -> [w160]
                tunnel: [w154] -> w149 mode=indexing
                i -> [w161]
                # "use only value at index \"Pixel\""
                # "init array of size PIXEL\nwith value 100"
                n149 = global read "Globals.vi" "PIXEL"() -> (w159:u32)
                n150 = Initialize Array(100, w159) -> (w157:i32[])
                n151 = call "ReturnFrame.vi"("Data Values In"=w157, "curr_nob"=w160, "curr_nos"=w161, "Drv"=1) -> ("Data Values Out"=w156:u16[])  [unwired: 1 in]
                n152 = Index Array(array=w156, index="Pixel") -> (element=w154:u16)
              }
              n153 = Delete From Array(array=w149, length=10, index=0) -> (array with subset deleted=w148:u16[])  [unwired: 1 out]
            }
            n154 = call <vilib>:"Std Deviation and Variance.vi"("X"=w143) -> ("mean"=→"mean":dbl, "standard deviation"=→"tRMS":dbl)  [unwired: 1 in, 1 out]
          }
        }
      }
    }
  }
  n155 = property on="NOS" class="Slide (strict)"("DisabledEnum"=w1) -> ()  [unwired: 2 in, 2 out]
  n156 = property on="start" class="Bool (strict)"("DisabledEnum"=w1) -> ()  [unwired: 2 in, 2 out]
  n157 = property on="NOB" class="Slide (strict)"("DisabledEnum"=w1) -> ()  [unwired: 2 in, 2 out]
